vi "Get_Event_Type.vi"(1 "Event":cluster{string, string[], dbl[], dbl}) -> (0 "Event Type":T1(ring))   [LabVIEW 2011]
doc: "This VI returns an enumerated value designating whether the given event should wait for user input, block growth sequence execution, or act normally."
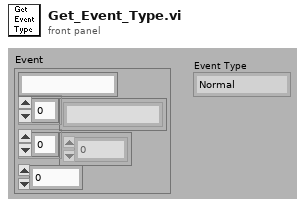
[diagram p1: front panel]
types:
  T1 = enum16{"Normal", "Blocking", "Wait for Input", "Loop"}
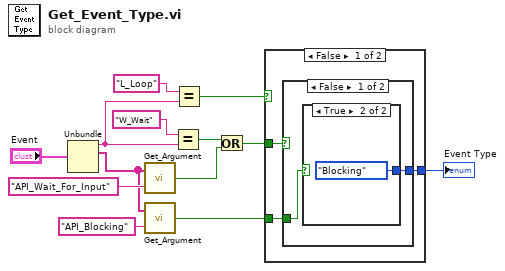
[diagram p0: block diagram]
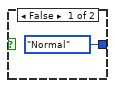
[diagram p2: hidden frame]
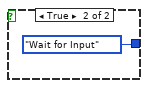
[diagram p3: hidden frame]
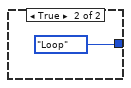
[diagram p4: hidden frame]
diagram:
  n1 = Unbundle("Event") -> (w4:string, w7:string[])  [unwired: 2 out]
  n2 = call "Get_Argument.vi"("Argument"="API_Wait_For_Input", "Argument List"=w7) -> ("Enabled"=w9:bool)
  n3 = call "Get_Argument.vi"("Argument"="API_Blocking", "Argument List"=w7) -> ("Enabled"=w5:bool)
  n4 = Equal?(x="W_Wait", y=w4) -> (x = y?=w11:bool)
  n5 = Equal?(x="L_Loop", y=w4) -> (x = y?=w2:bool)
  n6 = Or(x=w11, y=w9) -> (x .or. y?=w8:bool)
  n7 = case shown="False" w2 {
    tunnel: w8 -> [w16 _]
    tunnel: w5 -> [w15 _]
    tunnel: [w14 T1."Loop" ("Event Type")] -> w1
    frame False {
      n8 = case shown="False" w16 {
        tunnel: w15 -> [w18 _]
        tunnel: [w17 T1."Wait for Input" ("Event Type")] -> w14
        frame False {
          n9 = case shown="True" w18 {
            tunnel: [T1."Normal" ("Event Type") T1."Blocking" ("Event Type")] -> w17
            frame False {
            }
            frame True {
            }
          }
        }
        frame True {
        }
      }
    }
    frame True {
    }
  }
  "Event Type" <- w1
